vi "Target Method.vi"(6 "Target outfile":path=path "C:/Users/RSG/Desktop/NI-Skywater-Test-Setup/target.csv", 7 "Algorithm":u16, 8 "error in (no error)":errorcluster, 9 "Algo Param":dbl[](array[numeric]), 10 "Write Target":dbl[](array[numeric]), 11 "IVI Refnum in":refnum<k15>) -> (0 "error out":errorcluster, 1 "final resistance (ohm)":dbl, 2 "final current (A)":dbl, 3 "IVI Refnum out":refnum<k15>)   [LabVIEW 2018]
uses:
  Globals.vi
  <vilib>/Utility/file.llb/Write Delimited Spreadsheet (DBL).vi
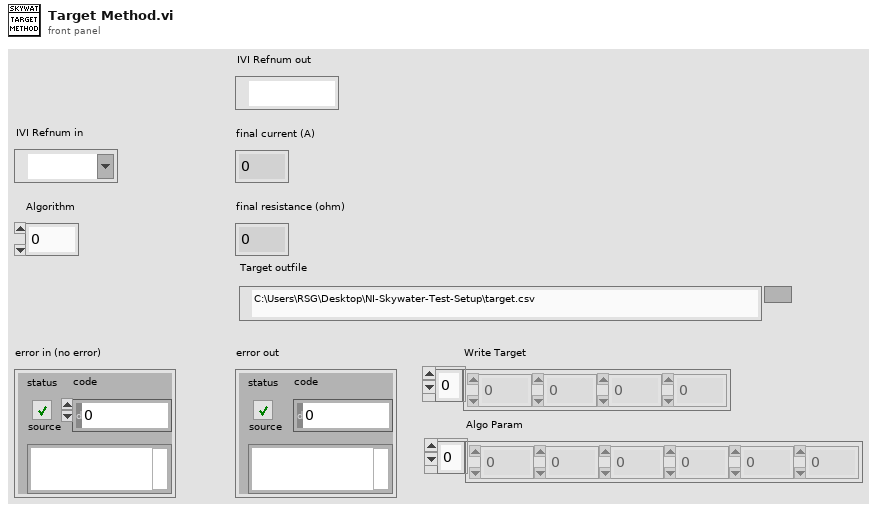
[diagram p1: front panel]
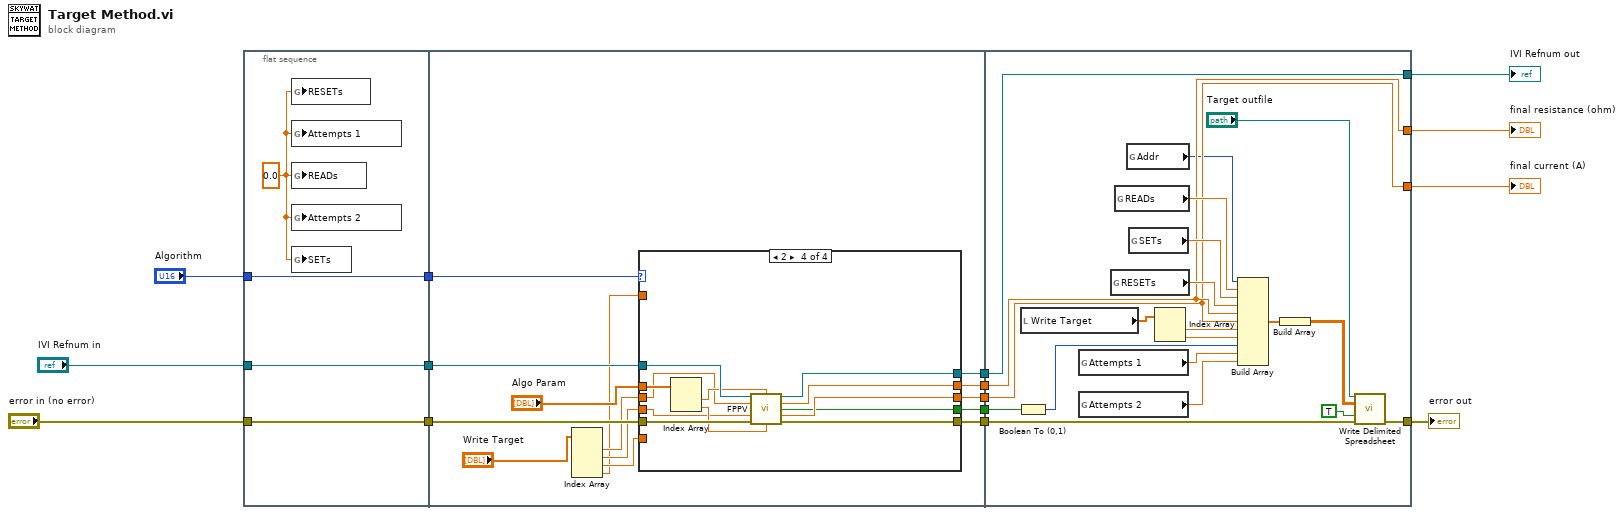
[diagram p0: block diagram]
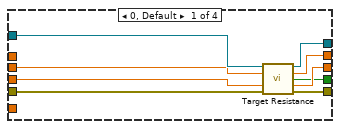
[diagram p2: hidden frame]
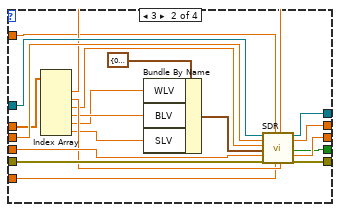
[diagram p3: hidden frame]
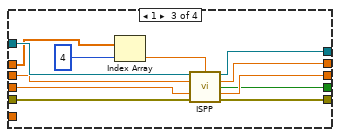
[diagram p4: hidden frame]
diagram:
  n1 = flat-sequence {
    tunnel: "error in (no error)" -> [w17]
    tunnel: "IVI Refnum in" -> [w18]
    tunnel: "Algorithm" -> [w19]
    tunnel: [w19] -> w4
    tunnel: [w18] -> w3
    tunnel: [w17] -> w2
    tunnel: [w32] -> w10
    tunnel: [w31] -> w9
    tunnel: [w30] -> w8
    tunnel: [w29] -> w7
    tunnel: w4 -> [w33]
    tunnel: w3 -> [w28]
    tunnel: w2 -> [w27]
    tunnel: [w26] -> w1
    tunnel: [w106] -> w13
    tunnel: [w95] -> w14
    tunnel: [w97] -> w5
    tunnel: [w98] -> w6
    tunnel: w10 -> [w98]
    tunnel: w9 -> [w97]
    tunnel: w8 -> [w96]
    tunnel: w7 -> [w106]
    tunnel: w1 -> [w93]
    frame #0 {
      w16 = 0.0 ("READs")
      n2 = global write "Globals.vi" "RESETs"(w16) -> ()
      n3 = global write "Globals.vi" "Attempts 1"(w16) -> ()
      n4 = global write "Globals.vi" "READs"(w16) -> ()
      n5 = global write "Globals.vi" "Attempts 2"(w16) -> ()
      n6 = global write "Globals.vi" "SETs"(w16) -> ()
    }
    frame #1 {
      n7 = Index Array(array="Write Target") -> (element #1=w23:dbl, element #2=w22:dbl, element #3=w21:dbl, element #4=w20:dbl)  [unwired: 4 in]
      n8 = case shown="2" w33 {
        tunnel: w27 -> [w42 w59 w74 w86]
        tunnel: w28 -> [w41 w62 w73 w85]
        tunnel: [w40 w61 w72 w84] -> w29
        tunnel: [w39 w60 w71 w83] -> w30
        tunnel: [w38 w57 w70 w82] -> w31
        tunnel: [w37 w58 w69 w81] -> w32
        tunnel: [w36 w56 w68 w80] -> w26
        tunnel: "Algo Param" -> [_ w53 w65 w79]
        tunnel: w23 -> [w35 w55 w64 w76]
        tunnel: w22 -> [w34 w54 w63 w75]
        tunnel: w21 -> [_ w43 _ _]
        tunnel: w20 -> [_ w44 _ _]
        frame 0, Default {
          n9 = call "Target Resistance.vi"("instrument handle"=w41, "Lower resistance (ohm)"=w35, "Upper resistance (ohm)"=w34, "error in (no error)"=w42) -> ("instrument handle out"=w40:refnum<k15>, "final resistance (ohm)"=w37:dbl, "target hit?"=w36:bool, "final current (A)"=w38:dbl, "error out"=w39:errorcluster)  [unwired: 4 in, 3 out]
        }
        frame 3 {
          n10 = Index Array(array=w53) -> (element #1=w51:dbl, element #2=w50:dbl, element #3=w49:dbl, element #4=w47:dbl, element #5=w46:dbl, element #6=w45:dbl)  [unwired: 6 in]
          n11 = Bundle By Name(cluster=cluster{"WLV":dbl, "BLV":dbl, "SLV":dbl} {"WLV"=0.06, "BLV"=0.4, "SLV"=0.8} ("Step Size"), "WLV"=w46, "BLV"=w47, "SLV"=w45) -> (w52:cluster{"WLV":dbl, "BLV":dbl, "SLV":dbl})
          n12 = call "SDR.vi"("instrument handle"=w62, "Rm (ohm)"=w55, "MLC SLV (V)"=w49, "Step Size"=w52, "RM (ohm)"=w54, "error in (no error)"=w59, "RMM (ohm)"=w44, "Rmm (ohm)"=w43, "MLC BLV (V)"=w51, "MLC WLV (V)"=w50) -> ("instrument handle out"=w61:refnum<k15>, "final resistance (ohm)"=w58:dbl, "target hit?"=w56:bool, "final current (A)"=w57:dbl, "error out"=w60:errorcluster)  [unwired: 2 in, 3 out]
        }
        frame 1 {
          n13 = Index Array(array=w65, index=4) -> (element=w67:dbl)
          n14 = call "ISPP.vi"("instrument handle"=w73, "Step size"=w67, "Lower resistance (ohm)"=w64, "Upper resistance (ohm)"=w63, "error in (no error)"=w74) -> ("instrument handle out"=w72:refnum<k15>, "final resistance (ohm)"=w69:dbl, "target hit?"=w68:bool, "final current (A)"=w70:dbl, "error out"=w71:errorcluster)  [unwired: 3 in, 3 out]
        }
        frame 2 {
          n15 = Index Array(array=w79) -> (element #1=w78:dbl, element #2=w77:dbl)  [unwired: 2 in]
          n16 = call "FPPV.vi"("instrument handle"=w85, "MLC BLV (V)"=w78, "Lower resistance (ohm)"=w76, "Upper resistance (ohm)"=w75, "error in (no error)"=w86, "MLC WLV (V)"=w77) -> ("instrument handle out"=w84:refnum<k15>, "final resistance (ohm)"=w81:dbl, "target hit?"=w80:bool, "final current (A)"=w82:dbl, "error out"=w83:errorcluster)  [unwired: 2 in, 3 out]
        }
      }
    }
    frame #2 {
      n17 = Boolean To (0,1)(Boolean=w93) -> (0, 1=w92:i16)
      n18 = local read "Write Target"() -> (w87:dbl[])
      n19 = global read "Globals.vi" "Attempts 1"() -> (w91:dbl)
      n20 = global read "Globals.vi" "Attempts 2"() -> (w90:dbl)
      n21 = global read "Globals.vi" "RESETs"() -> (w104:dbl)
      n22 = global read "Globals.vi" "READs"() -> (w102:dbl)
      n23 = global read "Globals.vi" "Addr"() -> (w94:i32)
      n24 = global read "Globals.vi" "SETs"() -> (w103:dbl)
      n25 = Index Array(array=w87) -> (element #1=w89:dbl, element #2=w88:dbl)  [unwired: 2 in]
      n26 = Build Array(w94, w102, w103, w104, w98, w97, w89, w88, w92, w91, w90) -> (w101:dbl[])
      n27 = Build Array(w101) -> (w100:dbl[][])
      n28 = call-poly <vilib>:"Write Delimited Spreadsheet.vi"("file path (dialog if empty)"="Target outfile", "2D data"=w100, "append to file? (new file:F)"=TRUE, "error in (no error)"=w96) -> ("error out"=w95:errorcluster)  [unwired: 10 in, 1 out]
    }
  }
  "final resistance (ohm)" <- w6
  "final current (A)" <- w5
  "error out" <- w14
  "IVI Refnum out" <- w13
